vi "SWERVE_DRIVE_GLOBALS.vi"() -> ()   [LabVIEW 2019]
panel:
  out "GyroHeading_Radians":dbl format="%17.2f"
  out "Chassis vOmega Speed":dbl format="%17.3f"
  out "Chassis vY Speed":dbl format="%17.3f"
  out "Chassis vX Speed":dbl format="%17.3f"
  out "Mod Speed Err":dbl[](array[numeric]) format="%17.3f"
  out "Mod Wheel Out":dbl[](array[numeric]) format="%17.3f"
  out "Mod Speed Act":dbl[](array[numeric]) format="%17.3f"
  out "Mod Speed Dmd":dbl[](array[numeric]) format="%17.3f"
  out "Mod Swerve in Deadband":bool
  out "Mod Swerve On Targ":bool[](array[boolean])
  out "Mod Swerve Err":dbl[](array[numeric]) format="%17.3f"
  out "Mod Swerve Out":dbl[](array[numeric]) format="%17.3f"
  out "Mod Angle Act":dbl[](array[numeric]) format="%17.3f"
  out "Mod Angle Dmd":dbl[](array[numeric]) format="%17.3f"
  out "Orientation Correct CO":dbl format="%17.3f"
  out "Orientation Angle Error_Rad":dbl format="%17.3f"
  out "Chassis vOmega Dmd":dbl format="%17.3f"
  out "Chassis vY Dmd":dbl format="%17.3f"
  out "Chassis vX Dmd":dbl format="%17.3f"
  out "Orientation Angle Dmd_Rad":dbl format="%17.3f"
  out "Drv Omega Vel Dmd":dbl format="%17.3f"
  out "Drv Y Vel Dmd":dbl format="%17.3f"
  out "Drv X Vel Dmd":dbl format="%17.3f"
  # "DIAGNOSTIC\nDATA"
  # "SWERVE DRIVE\nDEMANDS\nSPEED AND ORIENTATION"
  # "Sensor\nReadings\nand calcs"
  # "Module Drive\nSpeed"
  # "Module \nPositioning"
  # "Overall Chassis Dmd\nafter orientation correction"
  # "Orientation Correction data"
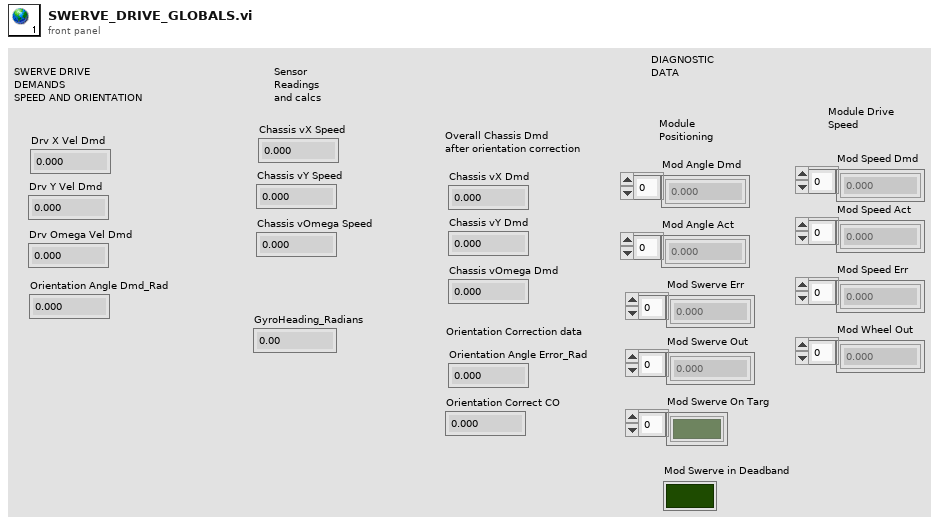
[diagram p1: front panel]
diagram:
